vi "Calculate TCP Server Port from GD ID.vi"(8 "error in (no error)":errorcluster, 11 "GD ID":string) -> (0 "error out":errorcluster, 3 "Port":u16)   [LabVIEW 2026, in "TALOS.lvlib"]
uses:
  TALOS.lvlib
  Ancestor/Ancestor/Ancestor.lvclass/Ancestor.ctl
  <vilib>/AdvancedString/Delimited String to 1D String Array (string).vi
  <vilib>/Utility/error.llb/Trim Whitespace (string).vi
  a3c4f305-f424-4c18-8907-55319b851364.vi
  2a529e7d-bc36-416e-93c6-8ccdf5b6dfb1.vi
  Circus Config Param - Core.vi
  <vilib>/Utility/error.llb/Trim Whitespace One-Sided.vi
  2a529e7d-bc36-416e-93c6-8ccdf5b6dfb1.vi/d4db2432-cc9c-482c-8957-dac855435ef6.vi
  2a529e7d-bc36-416e-93c6-8ccdf5b6dfb1.vi/86fbf154-bd7b-49a2-8ab2-a837b2a95f24.vi
  2a529e7d-bc36-416e-93c6-8ccdf5b6dfb1.vi/3b95b01e-1ec2-4565-bcd9-7606a5281010.vi
  2a529e7d-bc36-416e-93c6-8ccdf5b6dfb1.vi/96a08935-737a-44b2-979c-a81d56408f7e.vi
  FGV/Error Memory/Get Error Description.vi
  Get PC name.vi
  Ancestor/Ancestor/Read ID.vi
  Get Class Name.vi
  <vilib>/Utility/error.llb/Clear Errors.vi
  Circus Root Path.vi
  TALOS Config Param.vi
  2a529e7d-bc36-416e-93c6-8ccdf5b6dfb1.vi/d4db2432-cc9c-482c-8957-dac855435ef6.vi/6eaecd13-6e48-4772-a921-b51ebdf84d88.vi
  2a529e7d-bc36-416e-93c6-8ccdf5b6dfb1.vi/d4db2432-cc9c-482c-8957-dac855435ef6.vi/d2d5f2b7-06f4-47f6-971c-049c3fdbb653.vi
  2a529e7d-bc36-416e-93c6-8ccdf5b6dfb1.vi/3b95b01e-1ec2-4565-bcd9-7606a5281010.vi/6eaecd13-6e48-4772-a921-b51ebdf84d88.vi
  2a529e7d-bc36-416e-93c6-8ccdf5b6dfb1.vi/3b95b01e-1ec2-4565-bcd9-7606a5281010.vi/d2d5f2b7-06f4-47f6-971c-049c3fdbb653.vi
  2a529e7d-bc36-416e-93c6-8ccdf5b6dfb1.vi/96a08935-737a-44b2-979c-a81d56408f7e.vi/6eaecd13-6e48-4772-a921-b51ebdf84d88.vi
  2a529e7d-bc36-416e-93c6-8ccdf5b6dfb1.vi/96a08935-737a-44b2-979c-a81d56408f7e.vi/d2d5f2b7-06f4-47f6-971c-049c3fdbb653.vi
  FGV/Error Memory/Error Memory Core.vi
  FGV/Error Memory/Error Crt Lvl checker.vi
  FGV/Error Memory/Error Memory Core.vi/40c8088d-b597-4017-91af-faa98e00292e.vi
  FGV/Error Memory/Error Memory Core.vi/d4a3ab98-063c-4e44-b43d-fbdcfe6c2be2.vi
  Global Memory.vi
  <vilib>/Utility/LVClass/Get LV Class Name.vi
  Is in Packed Library.vi
  TALOS Root path.vi
  Read CSV worksheet.vi
  Global Constants.vi
  <vilib>/Utility/error.llb/General Error Handler.vi
  <vilib>/Utility/config.llb/Open Config Data.vi
  <vilib>/Utility/config.llb/Get Section Names.vi
  <vilib>/Utility/config.llb/Get Key Names.vi
  <vilib>/Utility/config.llb/Read Key.vi
  <vilib>/Utility/config.llb/Read Key (String).vi
  <vilib>/Utility/config.llb/Close Config Data.vi
  Ancestor/Ancestor/Ancestor.lvclass
  <vilib>/Comparison/Equal/Equal Functor/Equal Functor.lvclass
  <vilib>/Comparison/Less/Less Functor/Less Functor.lvclass
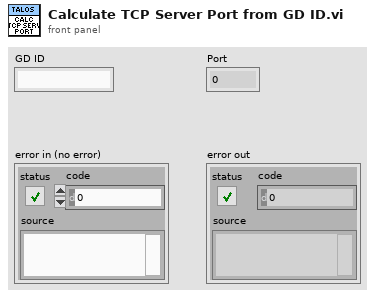
[diagram p1: front panel]
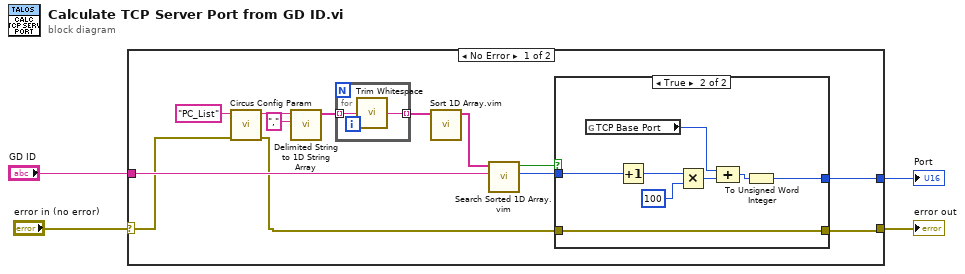
[diagram p0: block diagram]
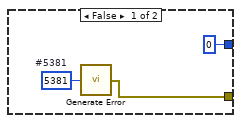
[diagram p2: hidden frame]
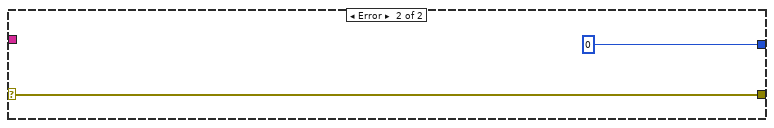
[diagram p3: hidden frame]
diagram:
  n1 = case shown="No Error" "error in (no error)" {
    selector: "error in (no error)" -> [w8 w31]
    tunnel: "GD ID" -> [w17 _]
    tunnel: [w16 u16 0] -> w3
    tunnel: [w5 w31] -> w1
    frame No Error {
      n2 = call "Circus Config Param.vi"("error in (no error)"=w8, "Parameter Name"="PC_List") -> ("error out"=w7:errorcluster, "Value"=w10:string)  [unwired: 8 in]
      n3 = call-poly <vilib>:"Delimited String to 1D String Array.vi"("delimiter"=",", "delimited string"=w10) -> ("string array"=w12:string[])  [unwired: 9 in]
      n4 = for {
        tunnel: w12 -> [w30] mode=indexing
        tunnel: [w29] -> w13 mode=indexing
        n5 = call-poly <vilib>:"Trim Whitespace.vi"("string"=w30) -> ("trimmed string"=w29:string)  [unwired: 1 in]
      }
      n6 = call "Sort 1D Array.vim"("unsorted array"=w13) -> ("sorted array"=w14:string[])  [unwired: 10 in]
      n7 = call "Search Sorted 1D Array.vim"("element"=w17, "sorted 1D array"=w14) -> ("nearest index"=w15:i32, "found?"=w6:bool)  [unwired: 8 in]
      n8 = case shown="True" w6 {
        tunnel: [u16 0 w28] -> w16
        tunnel: w15 -> [_ w22]
        tunnel: w7 -> [_ w21]
        tunnel: [w19 w21] -> w5
        frame False {
          w18 = 5381  # #5381
          n9 = call "Generate Error.vi"("Error Code"=w18) -> ("error out"=w19:errorcluster)  [unwired: 6 in]
        }
        frame True {
          n10 = global read "Global Constants.vi" "TCP Base Port"() -> (w25:u16)
          n11 = Increment(x=w22) -> (x+1=w23:i32)
          n12 = Multiply(x=w23, y=u16 100) -> (x*y=w26:i32)
          n13 = Compound Arithmetic op=ADD(w25, w26) -> (w27:i32)
          n14 = To Unsigned Word Integer(number=w27) -> (unsigned 16bit integer=w28:u16)
        }
      }
    }
    frame Error {
    }
  }
  "Port" <- w3
  "error out" <- w1
